vi "EmergencyStopAll.vi"() -> ()   [LabVIEW 2012]
uses:
  GenericDriveCommand.ctl
  DriveConfigGlobal.vi
  Anemometry/Anemometry Sub Vis/Globals/Trav_pos_global.vi
panel:
  out "Live Position":dbl[](array[numeric]) format="%.2f"
  in  "stop":bool
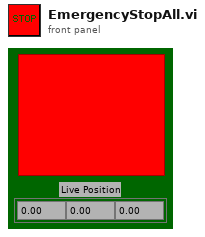
[diagram p1: front panel]
types:
  T1 = typedef "GenericDriveCommand.ctl" = string
  T2 = typedef "AxisConfigCluster.ctl" = cluster{"Channel Properties":T3, "Static Drive Configuration":T4}
  T3 = typedef "DriveProperties.ctl" = cluster{"Channel Name":string, "Vel. Default":dbl, "Acc. Default":dbl, "Vel. Max":dbl, "Vel. Min":dbl, "Acc. Max":dbl, "Acc. Min":dbl, "Pulses/unit":dbl, "Address":u8, "Pulse Offset":i32, "Pos Tolerance":dbl, "Pulses/rev":dbl, "Backlash/Eng units":dbl, "Current Pos":dbl, "Ch Status":enum16{"Active", "Offline", "Simulate"}, "Port Name":string, "Axis Transform mode":string, "Metadata Ch Name":string, "Type":string}
  T4 = typedef "DriveStaticConfig.ctl" = cluster{"Correction Gain % (CG)":u16, "Dead Band (DB)":i32, "Dead Band Window (DW)":i32, "Encoder Resolution (ER)":i32, "Step Mode  (FSB)":u16, "Position Maintenance (FSC)":u16, "Stop on Stall (FSD)":u16, "Activate OP1 on stall (FSE)":u16, "Stop on Trigger 3 (FSF)":u16, "OP2 in Deadband (FSG)":u16, "Stall Detect (FSH)":u16, "Limit Disable (LD)":u16, "Motor Resolution (MR)":enum16{"200", "400", "1000", "2000", "4000", "5000", "10000", "12800", "18000", "20000", "21600", "25000", "25400", "25600", "36000", "50000", "278528", "425984", "507904", "614400", "655360", "819200", "1024000"}, "Limit Switch Sense (OSA)":u16, "Home Position (OSB)":u16, "Home Switch Sense (OSC)":u16, "Encoder Z for Home (OSD)":u16, "Reference edge of Home (OSH)":u16, "RS232 Echo Control (SSA)":u16, "Buffer at Limit (SSG)":u16, "Buffer at Stop (SSH)":u16, "Indexer Mode  (FSA)":u16, "Type":string, "ConfigString":string, "De Power Motor":enum16{"TRUE", "FALSE"}}
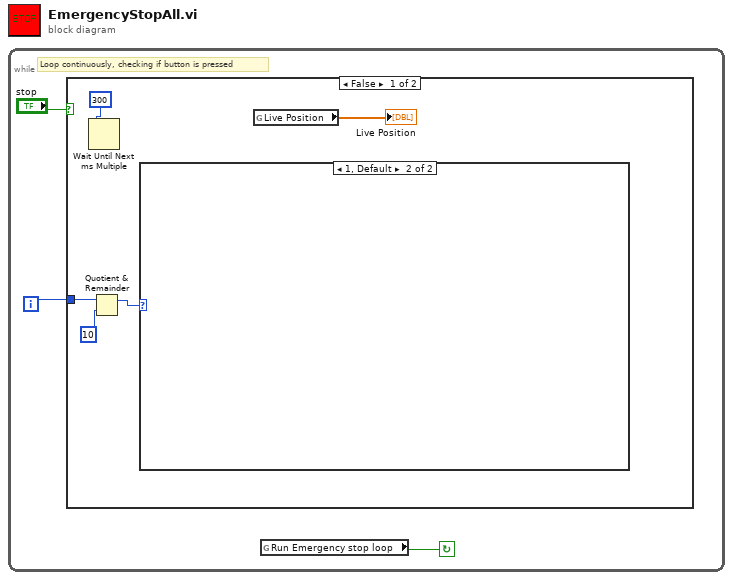
[diagram p0: block diagram]
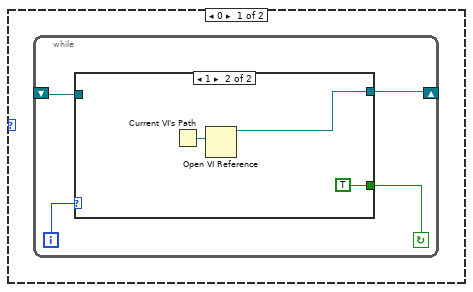
[diagram p2: hidden frame]
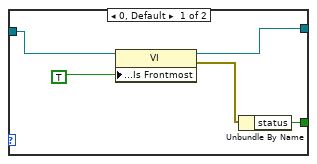
[diagram p3: hidden frame]
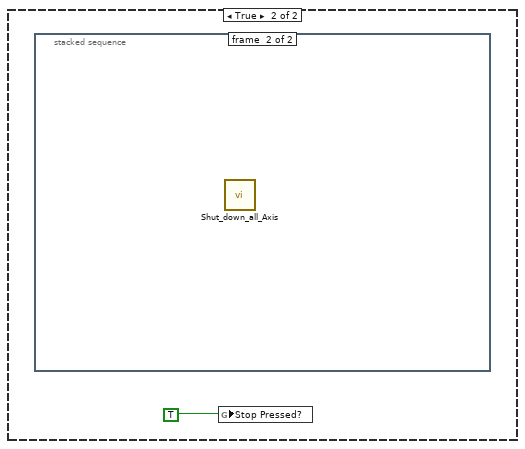
[diagram p4: hidden frame]
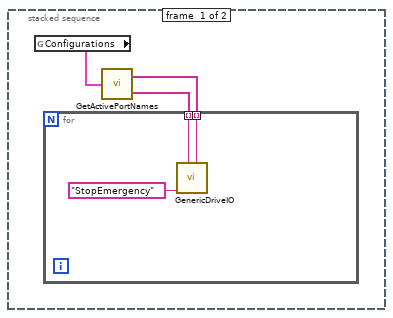
[diagram p5: hidden frame]
diagram:
  n1 = while {
    i -> [w1]
    stop <- w2 continue-if-true
    # "Loop continuously, checking if button is pressed"
    n2 = case shown="False" "stop" {
      tunnel: w1 -> [w7 _]
      frame False {
        n3 = Wait Until Next ms Multiple(millisecond multiple=300) -> ()  [unwired: 1 out]
        n4 = Quotient & Remainder(x=w7, y=10) -> (x-y*floor(x/y)=w5:i32)  [unwired: 1 out]
        n5 = case shown="1, Default" w5 {
          frame 0 {
            n6 = while {
              shift-left: _ -> [w12]
              shift-right: [w9] -> _
              i -> [w11]
              stop <- w10 continue-if-true
              n7 = case shown="1" w11 {
                tunnel: w12 -> [w16 _]
                tunnel: [w14 TRUE ("status")] -> w10
                tunnel: [w13 w19] -> w9
                frame 0, Default {
                  n8 = property class="VI"(reference=w16, "Front Panel Window:Is Frontmost"=TRUE) -> (reference out=w13:refnum<vi>, error out=w15:errorcluster)  [unwired: 1 in]
                  n9 = Unbundle By Name(w15) -> ("status"=w14:bool)
                }
                frame 1 {
                  n10 = Current VI's Path() -> (path=w20:path)
                  n11 = Open VI Reference(vi path=w20) -> (vi reference=w19:refnum<vi>)  [unwired: 5 in, 1 out]
                }
              }
            }
          }
          frame 1, Default {
          }
        }
        n12 = global read "Trav_pos_global.vi" "Live Position"() -> (→"Live Position":dbl[])
      }
      frame True {
        n13 = stacked-sequence {
          frame #0 {
            n14 = global read "DriveConfigGlobal.vi" "Configurations"() -> (w24:T2[])
            n15 = call "GetActivePortNames.vi"("Matched Configurations In"=w24) -> ("Port Name Array"=w23:string[], "Drive Type Array"=w22:string[])
            n16 = for {
              tunnel: w23 -> [w27] mode=indexing
              tunnel: w22 -> [w25] mode=indexing
              n17 = call "GenericDriveIO.vi"("GenericDriveCommand"=T1 "StopEmergency", "Type"=w25, "Port Name"=w27) -> ()  [unwired: 7 in, 2 out]
            }
          }
          frame #1 {
            n18 = call "Shut_down_all_Axis.vi"() -> ()  [unwired: 1 in]
          }
        }
        n19 = global write "DriveConfigGlobal.vi" "Stop Pressed?"(TRUE) -> ()
      }
    }
    n20 = global read "DriveConfigGlobal.vi" "Run Emergency stop loop"() -> (w2:bool)
  }
